vi "Add Wrapper to Library - Single Converter.vi"(11 "error in":errorcluster) -> (15 "error out":errorcluster)   [LabVIEW 2021, in "Converter.lvlib"]
uses:
  Converter.lvlib
  Path Functions/Path Functions.lvlib
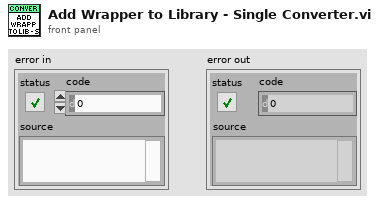
[diagram p1: front panel]
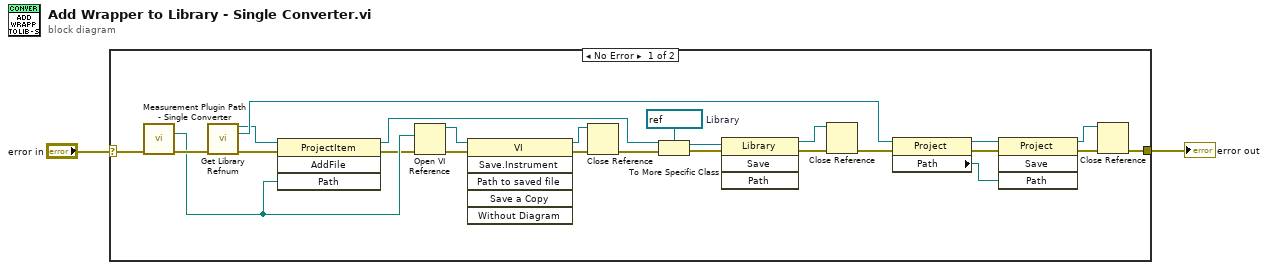
[diagram p0: block diagram]
diagram:
  n1 = case shown="No Error" "error in" {
    selector: "error in" -> [w17 w28]
    tunnel: [w24 w28] -> w2
    frame No Error {
      w13 = refnum<vi> refnum  # Library
      n2 = call "Measurement Plugin Path - Single Converter.vi"("error in"=w17) -> ("wrapper path"=w6:path, "error out"=w16:errorcluster)  [unwired: 2 in, 11 out]
      n3 = call "Get Library Refnum.vi"("error in"=w16) -> ("library refnum"=w14:refnum<vi>, "project:open"=w22:refnum<vi>, "error out"=w18:errorcluster)  [unwired: 12 in]
      n4 = invoke class="ProjectItem" method="AddFile"(reference=w14, error in=w18, "Path"=w6) -> (reference out=w10:refnum<vi>, error out=w4:errorcluster)  [unwired: 1 in, 2 out]
      n5 = Open VI Reference(vi path=w6, error in (no error)=w4) -> (vi reference=w5:refnum<vi>, error out=w3:errorcluster)  [unwired: 4 in]
      n6 = invoke class="VI" method="Save.Instrument"(reference=w5, error in=w3) -> (reference out=w7:refnum<vi>, error out=w8:errorcluster)  [unwired: 4 in, 4 out]
      n7 = Close Reference(reference=w7, error in (no error)=w8) -> (error out=w15:errorcluster)
      n8 = To More Specific Class(target class=w13, reference=w10, error in=w15) -> (specific class reference=w12:refnum<vi>, error out=w11:errorcluster)
      n9 = invoke class="Library" method="Save"(reference=w12, error in=w11) -> (reference out=w21:refnum<vi>, error out=w20:errorcluster)  [unwired: 2 in, 2 out]
      n10 = Close Reference(reference=w21, error in (no error)=w20) -> (error out=w19:errorcluster)
      n11 = property class="Project"(reference=w22, error in=w19) -> (reference out=w9:refnum<vi>, error out=w25:errorcluster, "Path"=w27:path)
      n12 = invoke class="Project" method="Save"(reference=w9, error in=w25, "Path"=w27) -> (reference out=w23:refnum<vi>, error out=w26:errorcluster)  [unwired: 1 in, 2 out]
      n13 = Close Reference(reference=w23, error in (no error)=w26) -> (error out=w24:errorcluster)
    }
    frame Error {
    }
  }
  "error out" <- w2
